vi "Eat.vi"(8 "error in (no error)":errorcluster, 11 "Philosopher in":refnum<class "Philosopher.lvclass">) -> (0 "error out":errorcluster, 3 "Philosopher out":refnum<class "Philosopher.lvclass">)   [LabVIEW 2023, in "Philosopher.lvlib" / "Philosopher.lvclass"]
uses:
  Philosopher.lvclass
  C:/Program Files (x86)/National Instruments/LabVIEW 2023/vi.lib/ActorFramework/Actor/Actor.lvclass
  Philosopher Messages/Timeout Hungry/Timeout Eating Msg.lvclass
  C:/Program Files (x86)/National Instruments/LabVIEW 2023/vi.lib/ActorFramework/Message/Message.lvclass
  <vilib>/ActorFramework/Actor/Actor.lvclass/Actor.ctl
  <vilib>/ActorFramework/Message Enqueuer/Message Enqueuer.lvclass/Message Enqueuer.ctl
  Philosopher.lvclass/Philosopher.ctl
  <vilib>/ActorFramework/Message Enqueuer/Init from Existing Queue.vi
  <vilib>/ActorFramework/Message Enqueuer/Message Enqueuer.lvclass
  <vilib>/ActorFramework/Actor/Actor.lvclass
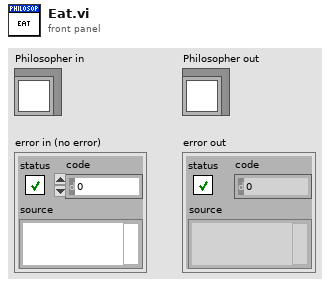
[diagram p1: front panel]
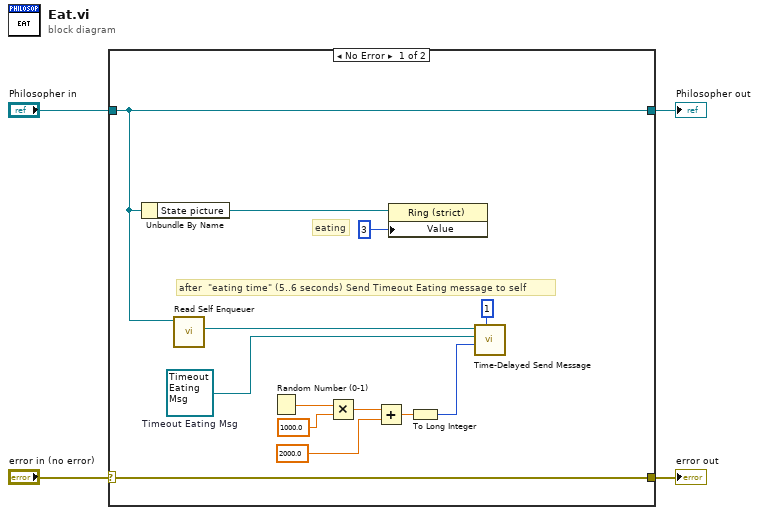
[diagram p0: block diagram]
diagram:
  n1 = case shown="No Error" "error in (no error)" {
    selector: "error in (no error)" -> [w17 w19]
    tunnel: [w17 w19] -> w3
    tunnel: [w16 w18] -> w1
    tunnel: "Philosopher in" -> [w16 w18]
    frame No Error {
      w13 = refnum<class "Timeout Eating Msg.lvclass"> refnum  # Timeout Eating Msg
      # "eating"
      # "after  \"eating time\" (5..6 seconds) Send Timeout Eating message to self"
      n2 = Unbundle By Name(w16) -> ("State picture"=w15:refnum<vi>)
      n3 = call <vilib>:"Read Self Enqueuer.vi"("Actor"=w16) -> ("Self Enqueuer"=w14:refnum<class "Message Enqueuer.lvclass">)  [unwired: 10 in]
      n4 = Random Number (0-1)() -> (number: 0 to 1=w11:dbl)
      n5 = Multiply(x=w11, y=1000.0) -> (x*y=w9:dbl)
      n6 = Add(x=w9, y=2000.0) -> (x+y=w7:dbl)
      n7 = property class="Ring (strict)"(reference=w15, "Value"=3) -> ()  [unwired: 1 in, 2 out]
      n8 = To Long Integer(number=w7) -> (32bit integer=w6:i32)
      n9 = call <vilib>:"Time-Delayed Send Message.vi"("# Copies (0 = infinite repeat)"=u32 1, "Milliseconds To Wait"=w6, "Message"=w13, "Message Enqueuer"=w14) -> ()  [unwired: 6 in, 2 out]
    }
    frame Error {
    }
  }
  "error out" <- w3
  "Philosopher out" <- w1
